vi "Driver Feedback Loop.vi"   [LabVIEW 2019]
uses:
  Shoot/Shooter Mode Type Def.ctl
  Climb/Climb Mode Type Def.ctl
  <vilib>/Rock Robotics/WPI/Utilities/WPI_GetSetVariantRefNum.vi
  Shoot/Shoot Global.vi
  Climb/Climb Global.vi
types:
  T1 = typedef "WPI_JoystickDevRef.ctl" = cluster{"Device":T2}
  T2 = typedef "WPI_JoystickDeviceEnum.ctl" = enum16{"USB 0", "USB 1", "USB 2", "USB 3", "USB 4", "USB 5"}
  T3 = typedef "WPI_MotorControlDeviceRef.ctl" = cluster{"DeviceStatus":errorcluster, "Type":T4, "PWM":cluster{"PWM Channel":T5, "DeadBand":T6}, "CAN":cluster{"Device Number":u8, "SetOutput VI Ref":variant, "GetOutput VI Ref":variant, "Enable VI Ref":variant, "Disable VI Ref":variant, "Data":variant}, "Invert":bool, "DIO PWM":cluster{"PWM \"Enable\" Channel":T5, "DIOChannel":T7, "PWM Rate":dbl}}
  T4 = typedef "WPI_MotorControlType.ctl" = enum16{"PWM", "CAN", "DIO PWM"}
  T5 = typedef "FPGA_DIOPWMChannel.ctl" = enum8{"PWM 0", "PWM 1", "PWM 2", "PWM 3", "PWM 4", "PWM 5", "PWM 6", "PWM 7", "PWM 8", "PWM 9", "PWM MXP 0", "PWM MXP 1", "PWM MXP 2", "PWM MXP 3", "PWM MXP 4", "PWM MXP 5", "PWM MXP 6", "PWM MXP 7", "PWM MXP 8", "PWM MXP 9", "Invalid"}
  T6 = typedef "WPI_PWMDeadband.ctl" = cluster{"Name":string, "maxPositivePwm":i32, "minPositivePwm":i32, "centerPwm":i32, "maxNegativePwm":i32, "minNegativePwm":i32, "angularRange":u16}
  T7 = typedef "FPGA_DIOChannel.ctl" = enum8{"DIO 0", "DIO 1", "DIO 2", "DIO 3", "DIO 4", "DIO 5", "DIO 6", "DIO 7", "DIO 8", "DIO 9", "DIO MXP 0", "DIO MXP 1", "DIO MXP 2", "DIO MXP 3", "DIO MXP 4", "DIO MXP 5", "DIO MXP 6", "DIO MXP 7", "DIO MXP 8", "DIO MXP 9", "DIO MXP 10", "DIO MXP 11", "DIO MXP 12", "DIO MXP 13", "DIO MXP 14", "DIO MXP 15", "SPI Port CS1", "SPI Port CS2", "SPI Port CS3", "SPI Port MISO", "SPI Port MOSI", "Invalid"}
  T8 = typedef "Climb Mode Type Def.ctl" = enum16{"Disabled", "Raw Throttle", "Auto Climb"}
  T9 = typedef "Shooter Mode Type Def.ctl" = enum16{"Disabled", "Raw Throttle", "Velocity Control"}
  T10 = typedef "Is command done typedef.ctl" = cluster{"Done?":bool, "Timestamp [ms]":dbl}
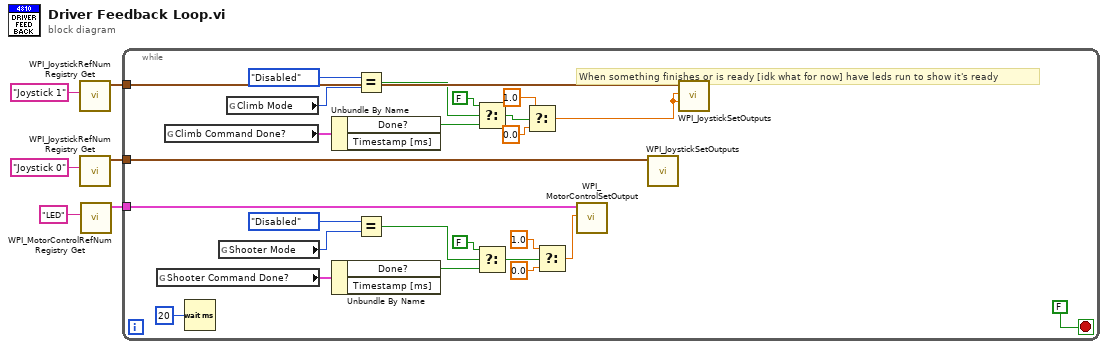
[diagram p0: block diagram]
diagram:
  n1 = call <vilib>:"WPI_JoystickRefNum Registry Get.vi"("refnum name"="Joystick 1") -> ("JoystickDevRef"=w5:T1)  [unwired: 9 in, 1 out]
  n2 = call <vilib>:"WPI_JoystickRefNum Registry Get.vi"("refnum name"="Joystick 0") -> ("JoystickDevRef"=w6:T1)  [unwired: 9 in, 1 out]
  n3 = call <vilib>:"WPI_MotorControlRefNum Registry Get.vi"("refnum name"="LED") -> ("MotorControlDevRef"=w1:T3)  [unwired: 9 in, 1 out]
  n4 = while {
    tunnel: w6 -> [w29]
    tunnel: w5 -> [w28]
    tunnel: w1 -> [w18]
    stop <- FALSE stop-if-true
    # "When something finishes or is ready [idk what for now] have leds run to show it's ready"
    n5 = global read "Shoot Global.vi" "Shooter Command Done?"() -> (w25:T10)
    n6 = global read "Climb Global.vi" "Climb Command Done?"() -> (w16:T10)
    n7 = Wait (ms)(milliseconds to wait=u32 20 ("millisecond timer value")) -> ()  [unwired: 1 out]
    n8 = global read "Shoot Global.vi" "Shooter Mode"() -> (w26:T9)
    n9 = global read "Climb Global.vi" "Climb Mode"() -> (w13:T8)
    n10 = Unbundle By Name(w16) -> ("Done?"=w11:bool)  [unwired: 1 out]
    n11 = Unbundle By Name(w25) -> ("Done?"=w22:bool)  [unwired: 1 out]
    n12 = Equal?(x=Climb_Mode_Type_Def."Disabled" ("Climb Mode"), y=w13) -> (x = y?=w12:bool)
    n13 = Equal?(x=Shooter_Mode_Type_Def."Disabled" ("Shooter Mode"), y=w26) -> (x = y?=w24:bool)
    n14 = Select(t=FALSE, s=w12, f=w11) -> (s? t:f=w9:bool)
    n15 = Select(t=FALSE, s=w24, f=w22) -> (s? t:f=w21:bool)
    n16 = Select(t=sgl 1.0 ("Left Rumble"), s=w9, f=sgl 0.0 ("Left Rumble")) -> (s? t:f=w7:sgl)
    n17 = Select(t=1.0, s=w21, f=0.0) -> (s? t:f=w17:dbl)
    n18 = call <vilib>:"WPI_MotorControlSetOutput.vi"("Output"=w17, "MotorControlDevRef"=w18) -> ()  [unwired: 7 in, 3 out]
    n19 = call <vilib>:"WPI_JoystickSetOutputs.vi"("JoystickDevRef"=w29) -> ()  [unwired: 9 in, 2 out]
    n20 = call <vilib>:"WPI_JoystickSetOutputs.vi"("Right Rumble"=w7, "Left Rumble"=w7, "JoystickDevRef"=w28) -> ()  [unwired: 7 in, 2 out]
  }
